vi "MALT BytesSwap.vi"(3 "In":string="A1F7149C") -> (1 "Out":string="9C14F7A1")   [LabVIEW 2018, in "AltonTech MALT200817.lvlib"]
uses:
  AltonTech MALT200817.lvlib
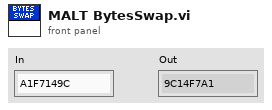
[diagram p1: front panel]
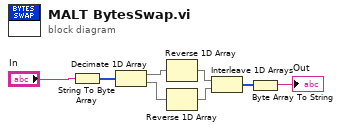
[diagram p0: block diagram]
diagram:
  n1 = String To Byte Array(string="In") -> (unsigned byte array=w7:u8[])
  n2 = Decimate 1D Array(w7) -> (w6:u8[], w5:u8[])
  n3 = Reverse 1D Array(array=w6) -> (reversed array=w4:u8[])
  n4 = Reverse 1D Array(array=w5) -> (reversed array=w3:u8[])
  n5 = Interleave 1D Arrays(w4, w3) -> (w2:u8[])
  n6 = Byte Array To String(unsigned byte array=w2) -> (string=→"Out":string)
